vi "ConvertPositions.vi"(0 "Input X":dbl, 1 "Input Y":dbl, 2 "error in":errorcluster) -> (3 "X":dbl, 4 "Y":dbl, 5 "concatenated string":string, 6 "error out":errorcluster)   [LabVIEW 2019]
panel:
  out "error out 2":errorcluster
  in  "MicronsPerPixel":dbl=0.6823
  in  "NPixelsY":dbl=2048.0
  in  "NPixelsX":dbl=2448.0
  in  "FileIn":path=path "C:/Users/TTUHEP/Documents/LabVIEW/GantryPrograms/Configs/OffsetsConstants.json"
  in  "ConversionType":T1(ring)
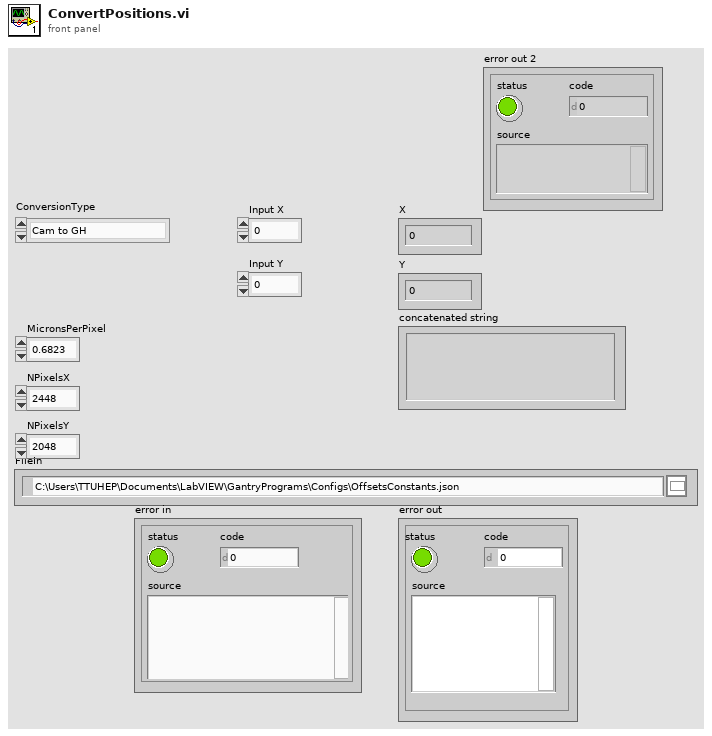
[diagram p1: front panel]
types:
  T1 = enum16{"Cam to GH", "Cam Pixel to GH", "GH to Cam", "Syringe to GH", "GH to Syringe", "Cam to Syringe", "Syringe to Cam"}
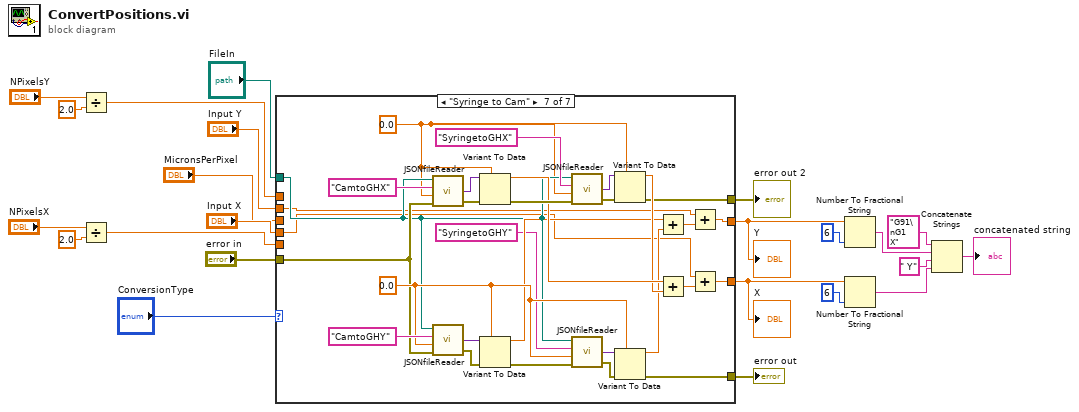
[diagram p0: block diagram]
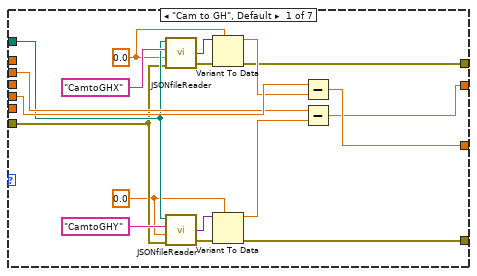
[diagram p2: hidden frame]
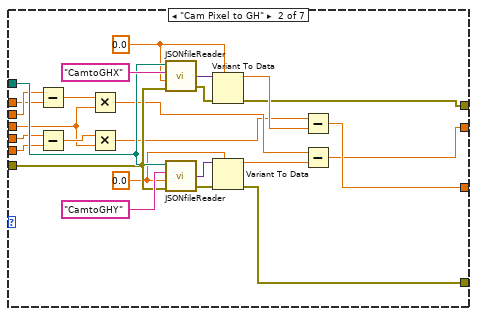
[diagram p3: hidden frame]
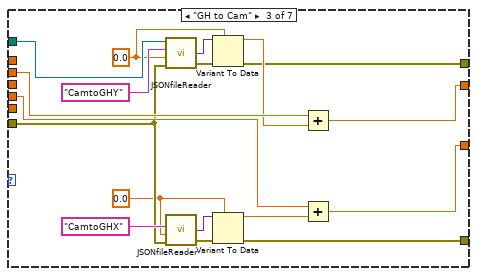
[diagram p4: hidden frame]
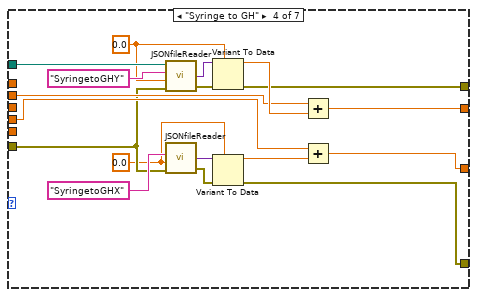
[diagram p5: hidden frame]
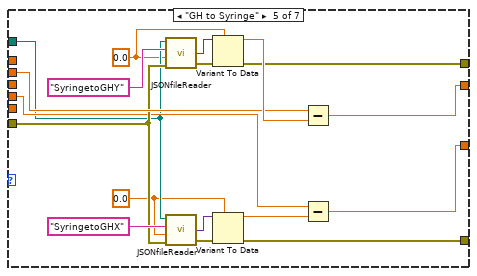
[diagram p6: hidden frame]
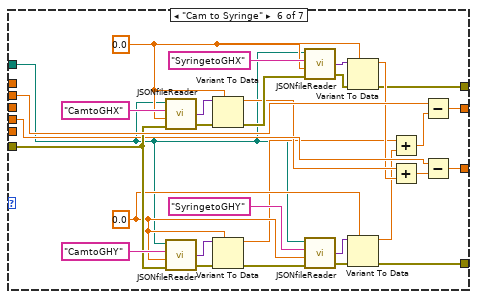
[diagram p7: hidden frame]
diagram:
  n1 = Divide(x="NPixelsY", y=2.0) -> (x/y=w13:dbl)
  n2 = Divide(x="NPixelsX", y=2.0) -> (x/y=w11:dbl)
  n3 = case shown="\"Syringe to Cam\"" "ConversionType" {
    tunnel: [w39 w57 w84 w93 w107 w134 w155] -> w8
    tunnel: [w38 w56 w83 w94 w112 w133 w156] -> w6
    tunnel: "Input X" -> [w41 w49 w82 w92 w109 w142 w153]
    tunnel: "Input Y" -> [w40 w53 w81 w91 w111 w144 w158]
    tunnel: "FileIn" -> [w29 w55 w72 w90 w108 w121 w160]
    tunnel: "error in" -> [w28 w54 w73 w89 w110 w143 w161]
    tunnel: [w27 w58 w70 w88 w106 w124 w152] -> w18
    tunnel: w13 -> [_ w52 _ _ _ _ _]
    tunnel: "MicronsPerPixel" -> [_ w46 _ _ _ _ _]
    tunnel: w11 -> [_ w48 _ _ _ _ _]
    tunnel: [w26 w44 w69 w87 w105 w125 w151] -> w1
    frame "Cam to GH", Default {
      w24 = 0.0
      w25 = 0.0
      n4 = call "JSONfileReader.vi"("error in"=w28, "Variant"=w25, "ItemName"="CamtoGHX", "FileIn"=w29) -> ("error out"=w36:errorcluster, "Data"=w37:variant)  [unwired: 1 out]
      n5 = call "JSONfileReader.vi"("error in"=w28, "Variant"=w24, "ItemName"="CamtoGHY", "FileIn"=w29) -> ("error out"=w34:errorcluster, "Data"=w35:variant)  [unwired: 1 out]
      n6 = Variant To Data(error in=w36, type=w25, Variant=w37) -> (data=w31:dbl, error out=w26:errorcluster)
      n7 = Variant To Data(error in=w34, type=w24, Variant=w35) -> (data=w32:dbl, error out=w27:errorcluster)
      n8 = Subtract(x=w41, y=w31) -> (x-y=w39:dbl)
      n9 = Subtract(x=w40, y=w32) -> (x-y=w38:dbl)
    }
    frame "Cam Pixel to GH" {
      w42 = 0.0
      w43 = 0.0
      n10 = Subtract(x=w53, y=w52) -> (x-y=w51:dbl)
      n11 = Subtract(x=w49, y=w48) -> (x-y=w47:dbl)
      n12 = Multiply(x=w51, y=w46) -> (x*y=w50:dbl)
      n13 = Multiply(x=w47, y=w46) -> (x*y=w45:dbl)
      n14 = call "JSONfileReader.vi"("error in"=w54, "Variant"=w43, "ItemName"="CamtoGHX", "FileIn"=w55) -> ("error out"=w65:errorcluster, "Data"=w66:variant)  [unwired: 1 out]
      n15 = call "JSONfileReader.vi"("error in"=w54, "Variant"=w42, "ItemName"="CamtoGHY", "FileIn"=w55) -> ("error out"=w63:errorcluster, "Data"=w64:variant)  [unwired: 1 out]
      n16 = Variant To Data(error in=w65, type=w43, Variant=w66) -> (data=w60:dbl, error out=w44:errorcluster)
      n17 = Variant To Data(error in=w63, type=w42, Variant=w64) -> (data=w61:dbl, error out=w58:errorcluster)
      n18 = Subtract(x=w45, y=w60) -> (x-y=w57:dbl)
      n19 = Subtract(x=w50, y=w61) -> (x-y=w56:dbl)
    }
    frame "GH to Cam" {
      w67 = 0.0
      w68 = 0.0
      n20 = call "JSONfileReader.vi"("error in"=w73, "Variant"=w67, "ItemName"="CamtoGHY", "FileIn"=w72) -> ("error out"=w75:errorcluster, "Data"=w76:variant)  [unwired: 1 out]
      n21 = call "JSONfileReader.vi"("error in"=w73, "Variant"=w68, "ItemName"="CamtoGHX") -> ("error out"=w77:errorcluster, "Data"=w79:variant)  [unwired: 1 in, 1 out]
      n22 = Variant To Data(error in=w75, type=w67, Variant=w76) -> (data=w74:dbl, error out=w69:errorcluster)
      n23 = Variant To Data(error in=w77, type=w68, Variant=w79) -> (data=w78:dbl, error out=w70:errorcluster)
      n24 = Add(x=w81, y=w74) -> (x+y=w83:dbl)
      n25 = Add(x=w82, y=w78) -> (x+y=w84:dbl)
    }
    frame "Syringe to GH" {
      w85 = 0.0
      w86 = 0.0
      n26 = call "JSONfileReader.vi"("error in"=w89, "Variant"=w85, "ItemName"="SyringetoGHY", "FileIn"=w90) -> ("error out"=w97:errorcluster, "Data"=w98:variant)  [unwired: 1 out]
      n27 = call "JSONfileReader.vi"("error in"=w89, "Variant"=w86, "ItemName"="SyringetoGHX") -> ("error out"=w99:errorcluster, "Data"=w101:variant)  [unwired: 1 in, 1 out]
      n28 = Variant To Data(error in=w97, type=w85, Variant=w98) -> (data=w96:dbl, error out=w87:errorcluster)
      n29 = Variant To Data(error in=w99, type=w86, Variant=w101) -> (data=w100:dbl, error out=w88:errorcluster)
      n30 = Add(x=w91, y=w96) -> (x+y=w94:dbl)
      n31 = Add(x=w92, y=w100) -> (x+y=w93:dbl)
    }
    frame "GH to Syringe" {
      w104 = 0.0
      w103 = 0.0
      n32 = call "JSONfileReader.vi"("error in"=w110, "Variant"=w104, "ItemName"="SyringetoGHY", "FileIn"=w108) -> ("error out"=w117:errorcluster, "Data"=w118:variant)  [unwired: 1 out]
      n33 = call "JSONfileReader.vi"("error in"=w110, "Variant"=w103, "ItemName"="SyringetoGHX", "FileIn"=w108) -> ("error out"=w119:errorcluster, "Data"=w120:variant)  [unwired: 1 out]
      n34 = Variant To Data(error in=w117, type=w104, Variant=w118) -> (data=w115:dbl, error out=w105:errorcluster)
      n35 = Variant To Data(error in=w119, type=w103, Variant=w120) -> (data=w114:dbl, error out=w106:errorcluster)
      n36 = Subtract(x=w111, y=w115) -> (x-y=w112:dbl)
      n37 = Subtract(x=w109, y=w114) -> (x-y=w107:dbl)
    }
    frame "Cam to Syringe" {
      w129 = 0.0
      w123 = 0.0
      n38 = call "JSONfileReader.vi"("error in"=w143, "Variant"=w123, "ItemName"="CamtoGHX", "FileIn"=w121) -> ("error out"=w149:errorcluster, "Data"=w150:variant)  [unwired: 1 out]
      n39 = call "JSONfileReader.vi"("error in"=w143, "Variant"=w129, "ItemName"="CamtoGHY", "FileIn"=w121) -> ("error out"=w147:errorcluster, "Data"=w148:variant)  [unwired: 1 out]
      n40 = Variant To Data(error in=w149, type=w123, Variant=w150) -> (data=w137:dbl, error out=w139:errorcluster)
      n41 = Variant To Data(error in=w147, type=w129, Variant=w148) -> (data=w122:dbl, error out=w128:errorcluster)
      n42 = call "JSONfileReader.vi"("error in"=w139, "Variant"=w123, "ItemName"="SyringetoGHX", "FileIn"=w121) -> ("error out"=w140:errorcluster, "Data"=w141:variant)  [unwired: 1 out]
      n43 = call "JSONfileReader.vi"("error in"=w128, "Variant"=w129, "ItemName"="SyringetoGHY", "FileIn"=w121) -> ("error out"=w131:errorcluster, "Data"=w132:variant)  [unwired: 1 out]
      n44 = Variant To Data(error in=w140, type=w123, Variant=w141) -> (data=w136:dbl, error out=w125:errorcluster)
      n45 = Variant To Data(error in=w131, type=w129, Variant=w132) -> (data=w130:dbl, error out=w124:errorcluster)
      n46 = Add(x=w122, y=w130) -> (x+y=w126:dbl)
      n47 = Add(x=w137, y=w136) -> (x+y=w135:dbl)
      n48 = Subtract(x=w144, y=w126) -> (x-y=w133:dbl)
      n49 = Subtract(x=w142, y=w135) -> (x-y=w134:dbl)
    }
    frame "Syringe to Cam" {
      w165 = 0.0
      w159 = 0.0
      n50 = call "JSONfileReader.vi"("error in"=w161, "Variant"=w159, "ItemName"="CamtoGHX", "FileIn"=w160) -> ("error out"=w179:errorcluster, "Data"=w180:variant)  [unwired: 1 out]
      n51 = call "JSONfileReader.vi"("error in"=w161, "Variant"=w165, "ItemName"="CamtoGHY", "FileIn"=w160) -> ("error out"=w177:errorcluster, "Data"=w178:variant)  [unwired: 1 out]
      n52 = Variant To Data(error in=w179, type=w159, Variant=w180) -> (data=w170:dbl, error out=w172:errorcluster)
      n53 = Variant To Data(error in=w177, type=w165, Variant=w178) -> (data=w163:dbl, error out=w164:errorcluster)
      n54 = call "JSONfileReader.vi"("error in"=w172, "Variant"=w159, "ItemName"="SyringetoGHX", "FileIn"=w160) -> ("error out"=w173:errorcluster, "Data"=w174:variant)  [unwired: 1 out]
      n55 = call "JSONfileReader.vi"("error in"=w164, "Variant"=w165, "ItemName"="SyringetoGHY", "FileIn"=w160) -> ("error out"=w167:errorcluster, "Data"=w168:variant)  [unwired: 1 out]
      n56 = Variant To Data(error in=w173, type=w159, Variant=w174) -> (data=w169:dbl, error out=w151:errorcluster)
      n57 = Variant To Data(error in=w167, type=w165, Variant=w168) -> (data=w166:dbl, error out=w152:errorcluster)
      n58 = Add(x=w163, y=w166) -> (x+y=w157:dbl)
      n59 = Add(x=w170, y=w169) -> (x+y=w154:dbl)
      n60 = Add(x=w158, y=w157) -> (x+y=w156:dbl)
      n61 = Add(x=w153, y=w154) -> (x+y=w155:dbl)
    }
  }
  "X" <- w8
  "Y" <- w6
  "error out" <- w18
  "error out 2" <- w1
  n62 = Number To Fractional String(number=w6, precision (6)=i16 6) -> (F-format string=w4:string)  [unwired: 2 in]
  n63 = Number To Fractional String(number=w8, precision (6)=i16 6) -> (F-format string=w3:string)  [unwired: 2 in]
  n64 = Concatenate Strings("G91\nG1 X", w4, " Y", w3) -> (→"concatenated string":string)
